vi "ArrayToExcel.vi"() -> ()   [LabVIEW 2020]
uses:
  <vilib>/Analysis/NI_AALBase.lvlib
panel:
  out "Tabla":string[][](array[string])
  out "Suma de Senos":dbl[][](graph)
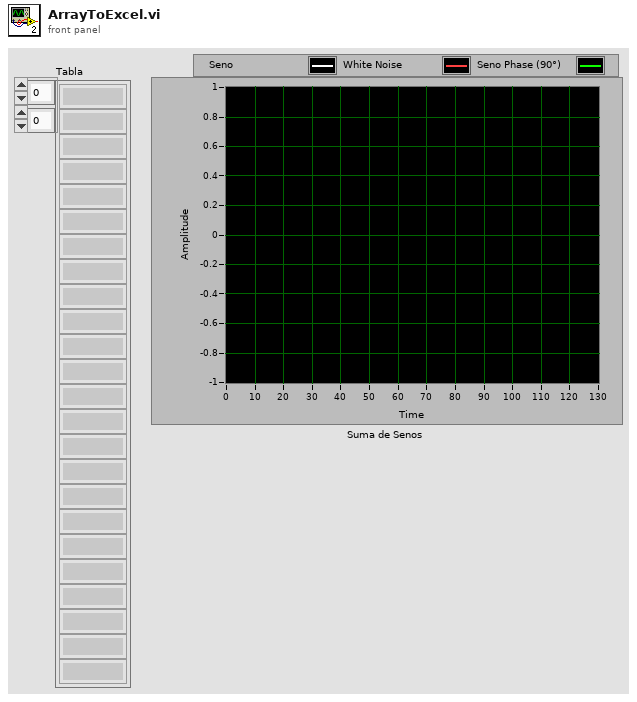
[diagram p1: front panel]
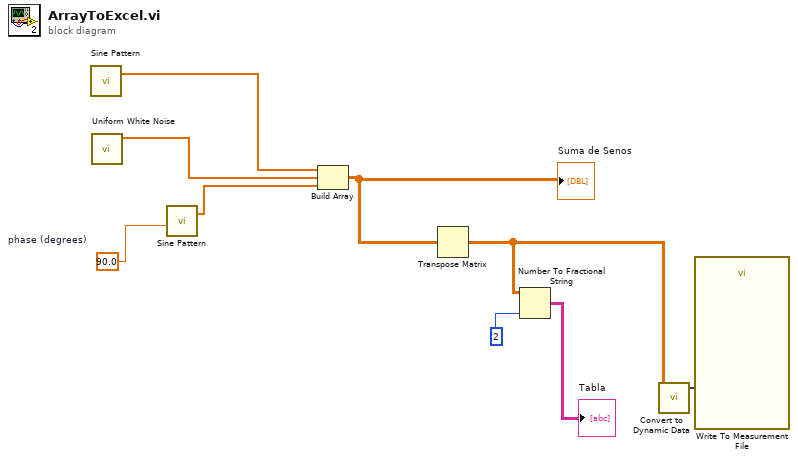
[diagram p0: block diagram]
diagram:
  w1 = 90.0  # phase (degrees)
  n1 = call <vilib>:"Sine Pattern.vi"() -> ("Sinusoidal Pattern"=w9:dbl[])  [unwired: 4 in, 1 out]
  n2 = call <vilib>:"Uniform White Noise.vi"() -> ("uniform white noise"=w2:dbl[])  [unwired: 10 in, 1 out]
  n3 = call <vilib>:"Sine Pattern.vi"("phase(degrees)"=w1) -> ("Sinusoidal Pattern"=w8:dbl[])  [unwired: 3 in, 1 out]
  n4 = Build Array "Build Array"(w9, w2, w8) -> (w6:dbl[][])
  "Suma de Senos" <- w6
  n5 = Transpose Matrix(1:w6) -> (0:w4:dbl[][])
  n6 = Number To Fractional String(number=w4, precision (6)=2) -> (F-format string=→"Tabla":string[][])  [unwired: 2 in]
  n7 = call "Convert to Dynamic Data"("2D Array"=w4) -> ("Dynamic Data Type"=w7:dynamicdata)  [unwired: 3 in]
  n8 = call "Write To Measurement File"("Signals"=w7) -> ()  [unwired: 16 in, 3 out]
